vi "Washing Machine Problem.vi"() -> ()   [LabVIEW 2016]
panel:
  out "Tank":dbl(slide) scale=0.0..100.0
  out "Motor":bool
  out "Thermometer":dbl(slide) scale=0.0..100.0
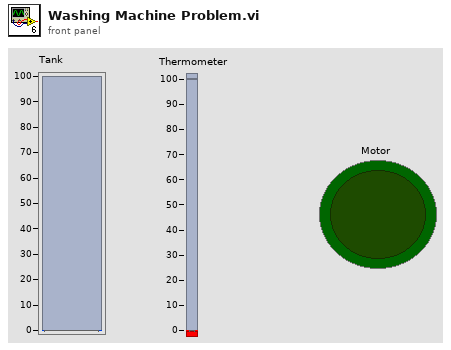
[diagram p1: front panel]
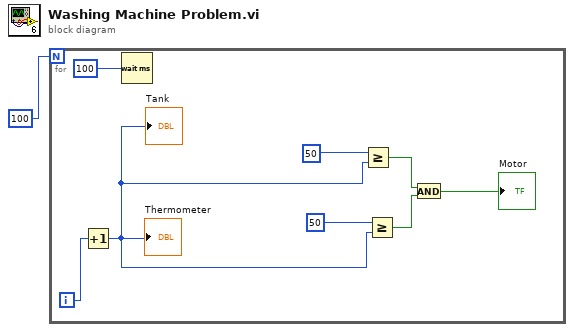
[diagram p0: block diagram]
diagram:
  n1 = for {
    N: 100 ("Numeric") -> [_]
    i -> [w9]
    n2 = Increment(x=w9) -> (x+1=w4:i32)
    "Thermometer" <- w4
    "Tank" <- w4
    n3 = Wait (ms)(milliseconds to wait=100) -> ()  [unwired: 1 out]
    n4 = Greater Or Equal?(x=50, y=w4) -> (x >= y?=w5:bool)
    n5 = Greater Or Equal?(x=50, y=w4) -> (x >= y?=w6:bool)
    n6 = And(x=w5, y=w6) -> (x .and. y?=→"Motor":bool)
  }
